vi "CSClassUtilities.TestClass.vi"() -> ()   [LabVIEW 2014]
doc: "Test VI for objects and classes.\n\nLicense Agreement for this software:\n\nCopyright (C) 2001 Dietrich Beck, Holger Brand, Mathias Richter\nGSI Helmholtzzentrum für Schwerionenforschung GmbH\nPlanckstraße 1\nD-64291 Darmstadt\nGermany\n\nContact: d.beck@gsi.de \n\nThis program is free software: you can redistribute it and/or modify it under the terms\nof the GNU General Public License as published by the Free Software Foundation, either\nversion 3 of the License, or (at your option) any later version.\n\nThis program is distributed in the hope that it will be useful, but WITHOUT ANY WARRANTY;\nwithout even the implied warranty of MERCHANTABILITY or FITNESS FOR A PARTICULAR PURPOSE. See the GNU General Public License for more details.\n\nYou should have received a copy of the GNU General Public License along with this program.\nIf not, see <http://www.gnu.org/licenses/>.\n\nFor all questions and ideas contact: d.beck@gsi.de\nLast update: 19-Nov-2010"
uses:
  CSClass/CS_Core/CSSystem/CoreDefs/CoreDefs.error_type.ctl
  CSClass/CS_Core/CSObj/CSObj.lvlib
  CSClass/CS_Core/CSSystem/CoreLib/CoreLib.lvlib
  CSClass/CS_Core/CAEObj/CAEObj.lvlib
  CSClass/CS_Core/NotifierObj/NotifierObj.lvlib
  CSClass/CS_Core/BaseProcess/BaseProcess.lvlib
  CSClass/CS_Core/SuperProc/SuperProc.lvlib
  CSClass/CS_Core/BaseGUI/BaseGUI.lvlib
  CSClass/CS_Core/ObjectInspector/ObjectInspector.lvlib
  CSClass/CS_Core/BaseSM/BaseSM.lvlib
  CSClass/CS_Core/CSSystem/CSSystemLib/CSSystemLib.lvlib
  CSClass/CS_Core/GUIs/GeneralObjectGUI/GeneralObjectGUI.lvlib
  CSClass/CS_Core/CSAccessSystem/CSAccessClient/CSAccessClient.lvlib
  CSClass/CS_Core/GUIs/GOGFrontPanel/GOGFrontPanel.lvlib
panel:
  in  "destroy all objects":bool
  in  "Expert Attr View":bool
  in  "TestProcCases":bool
  in  "Ping":bool
  in  "Object Classes":i32(listbox)=-1
  out "i attribute":variant=variant(cluster{"VI Refnum":refnum<vi>, "Front Panel Ref":refnum<vi>, "semaphore":refnum<k1>, "date of birth":u32} {"VI Refnum"=refnum, "Front Panel Ref"=refnum, "semaphore"=refnum, "date of birth"=511974648})
  out "Error":bool
  in  "Get Attribute":bool
  in  "Select Object":i32(listbox)=-1
  in  "Select Class":i32(listbox)=-1
  out "Error String":string="No Error"
  in  "Close FP":bool
  in  "Open FP":bool
  in  "Destroy":bool
  in  "object name":string
  in  "Create":bool
  in  "Exit":bool
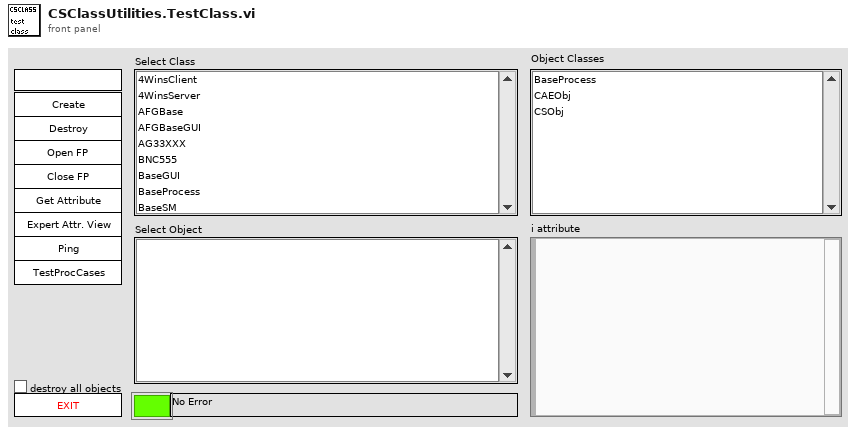
[diagram p1: front panel]
types:
  T1 = enum16{"simple", "synchronous", "asynchronous", "notification"}
  T2 = typedef "CoreDefs.error_type.ctl" = enum16{"no error", "can't load process", "can't unload process", "process does not exist", "can't install process", "can't remove process", "unknown function", "time out", "can't execute function", "duplicate queue name", "super not found", "caller queue invalid", "can't ping process", "unknown error", "VISA Error", "VISA timeout", "GPIB timeout", "GPIB error", "communication error", "data type mismatch", "can't read data from OPC server", "can't write data to OPC server", "OET error", "function not implemented", "process already exists", "invalid Shared Variable name", "error writing Shared Variable", "error reading Shared Variable", "invalid client name", "corrupt database", "unknown class", "call not authorized", "parameter out of range", "OET timeout: can't get data to modify", "invalid queue name", "requested operation incompatible with current state", "event undefined", "event disabled", "state undefined", "caller is not a friend", "EventBuilder: bad eventID", "EventBuilder: no DAQ devices", "a thread must not stop itself", "UNUSED ELEMENT4", "DiscArchiver: eventData incomplete", "DiscArchiver: eventData does not belong to run", "DiscArchiver: can't open file", "DiscArchiver: can't write to file", "DiscArchiver: available disc space low", "can't acquire semaphore", "error reading data from database", "notifier object is not existing", "can't register process", "can't unregister process", "illegal event type", "object disabled", "object already exists", "can't change state", "Instrument not found", "no connection to remote node", "invalid reference", "N/A", "UNUSED ELEMENT 1", "element not found", "illegal TCP/IP connection detected", "object does not exist", "invalid access ID", "unknown CS system", "invalid privilige", "unsupported data type", "unsupported server type", "IO server already exists", "Shared Variable already exists"}
  T3 = typedef "BaseGUI.lvlib/BaseGUI.i attribute.ctl" = cluster{"thread ref":refnum<vi>}
  T4 = typedef "BaseProcess.lvlib/BaseProcess.i attribute.ctl" = cluster{"EventStatus":string, "EventError":i32, "PresetEvtWatchD":i32, "PresetPdcWatchD":i32, "EventTimeout":i32, "PeriodicInterval":i32, "Interface":string[], "Address":string[], "Special":string[], "PeriodicError":i32, "PeriodicStatus":string, "SuperProc":string, "Descriptors":T5[], "CaseRef":refnum<vi>, "PdcRef":refnum<vi>, "Thread Ref":refnum<vi>, "eventErrorID":i32, "eventStatusID":i32, "periodicErrorID":i32, "periodicStatusID":i32, "pdcCtrID":i32}
  T5 = typedef "BaseProcess.lvlib/BaseProcess.descriptor definition.ctl" = cluster{"selector":string, "descriptor":T6}
  T6 = typedef "BaseProcess.lvlib/BaseProcess.descriptor string definition.ctl" = string
  T7 = typedef "BaseSM.lvlib/BaseSM.i attribute.ctl" = cluster{"stateError":i32, "stateStatus":string, "stateQuality":T8, "ProcStateRef":refnum<vi>, "thread ref":refnum<vi>, "actState":string, "reqState":string, "SMQueue":refnum<queue>, "stateErrorID":i32, "stateStatusID":i32}
  T8 = typedef "BaseSM.lvlib/BaseSM.stateQuality.ctl" = i16
  T9 = typedef "CAEObj.lvlib/CAEObj.i attribute.ctl" = cluster{"initialized":bool, "active":bool, "stop":bool, "evtCtrID":i32, "queue":T10, "selector":string[], "URL":string[], "commandID":i32[], "enable":bool[], "ignoreResID":bool[], "NotifyObj":refnum<vi>, "myAccessID":i32, "treeParentName":string, "myAccessIDID":i32, "treeParentAccessIDID":i32, "treeParentNameID":i32, "treeParentAccessIDRef":T11, "treeParentNameRef":T11, "threadRef":refnum<vi>}
  T10 = typedef "LVDimInterface.lvlib/LVDimInterface.queue type.ctl" = refnum<queue>
  T11 = typedef "LVDimInterface.lvlib/LVDimInterface.notifier type.ctl" = refnum<notifier>
  T12 = typedef "CSAccessClient.lvlib/CSAccessClient.i attribute.ctl" = cluster{"creatorRef":refnum<vi>, "actualTreeID":i32, "actualTreeRef":T11}
  T13 = typedef "CSObj.lvlib/CSObj.i attribute.ctl" = cluster{"VI Refnum":refnum<vi>, "Front Panel Ref":refnum<vi>, "semaphore":T14, "date of birth":dbl, "ageID":i32, "systemID":i32, "classID":i32, "conditionID":i32, "DefaultPanelType":u16}
  T14 = typedef "Semaphore RefNum" = refnum<k1>
  T15 = typedef "GeneralObjectGUI.lvlib/GeneralObjectGUI.i attribute.ctl" = cluster{"objects":T16[], "setting file":string, "fpElements":cluster{"busy":refnum<vi>, "status":refnum<vi>}, "accessClientRef":refnum<vi>, "ColumnWidth":u32[], "PanelBounds":T19}
  T16 = typedef "GeneralObjectGUI.lvlib/GeneralObjectGUI.object.ctl" = cluster{"name":string, "systemID":string, "AutoCreate":bool, "Enable":bool, "methods":T17[], "ActError":i32, "Tags":T18[]}
  T17 = typedef "GeneralObjectGUI.lvlib/GeneralObjectGUI.method.ctl" = cluster{"AutoExecute":bool, "Reset":bool, "Enable":bool, "Name":string, "Values":cluster{"descriptor":string, "value":string}[], "fp ref":refnum<vi>}
  T18 = typedef "GeneralObjectGUI.lvlib/GeneralObjectGUI.tag.ctl" = cluster{"name":string, "value":string}
  T19 = typedef "LVRectTypeDef.ctl" = cluster{"Left":i16, "Top":i16, "Right":i16, "Bottom":i16}
  T20 = typedef "GOGFrontPanel.lvlib/GOGFrontPanel.i attribute.ctl" = cluster{"GOGObject":string, "Object":string, "Method":string, "Descriptor":T6, "Input Descriptor":string, "Output Descriptor":string, "inputNames":string[], "outputNames":string[], "Values":cluster{"descriptor":string, "value":string}[]}
  T21 = typedef "NotifierObj.lvlib/NotifierObj.i attribute.ctl" = cluster{"associatedObjRef":refnum<vi>, "Notifiers":cluster{"Name":string, "Message":i8[], "Noti missed":i32, "Msg Sent":bool, "ref":T11}[], "commandIDs":i32[], "request stop":bool, "thread ref":refnum<vi>, "Enqueue at opposite":bool}
  T22 = typedef "ObjectInspector.lvlib/ObjectInspector.i attribute.ctl" = cluster{"ClassPaths":string[]}
  T23 = typedef "SuperProc.lvlib/SuperProc.i attribute.ctl" = cluster{"Proc Tbl":T24[]}
  T24 = typedef "SuperProc.lvlib/SuperProc.proc_tbl_type.ctl" = cluster{"Name":string, "Connections":i32, "Clients":string[], "EvtWDAlarmTime":u32, "PdcWDAlarmTime":u32, "PresetEvtWatchD":i32, "PresetPdcWatchD":i32, "i ref":refnum<vi>, "evtCounterRef":T11, "evtCounterID":i32, "pdcCounterRef":T11, "pdcCounterID":i32, "watchdogValue":i32, "watchdogID ":i32}
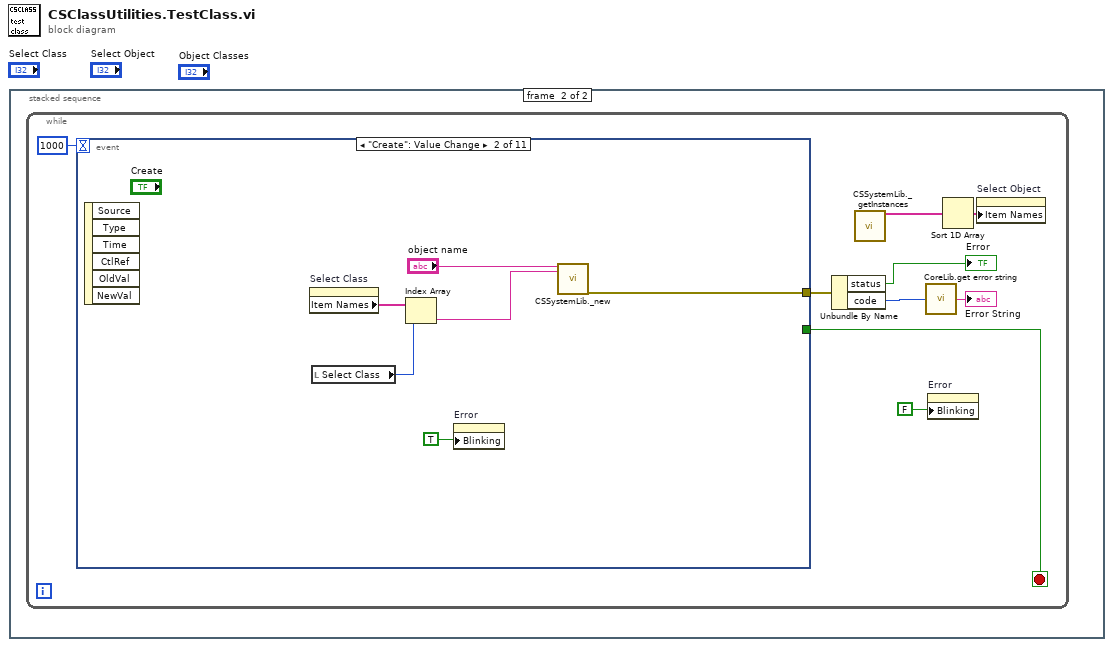
[diagram p0: block diagram]
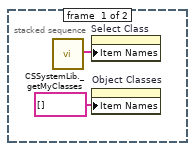
[diagram p2: hidden frame]
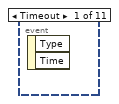
[diagram p3: hidden frame]
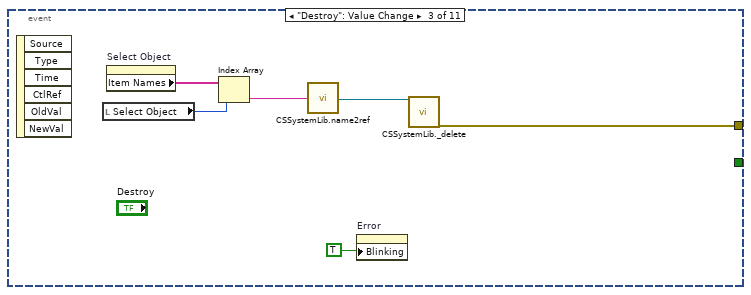
[diagram p4: hidden frame]
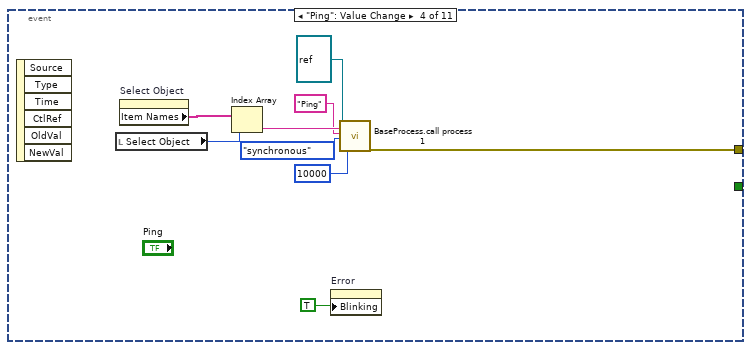
[diagram p5: hidden frame]
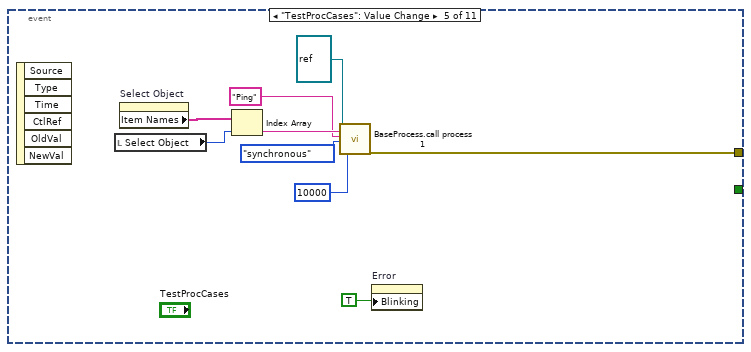
[diagram p6: hidden frame]
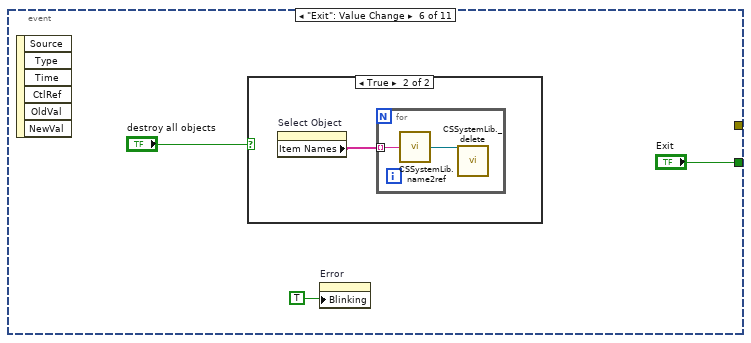
[diagram p7: hidden frame]
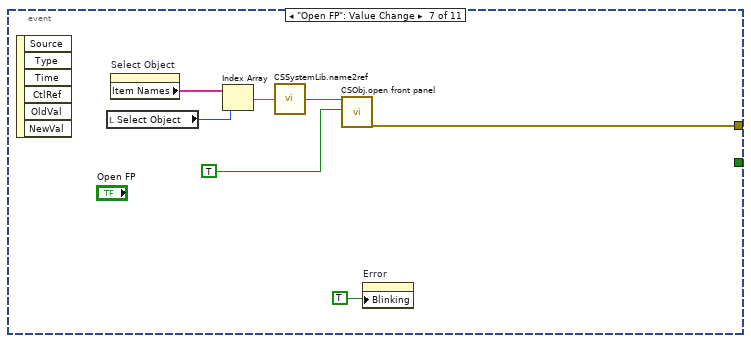
[diagram p9: hidden frame]
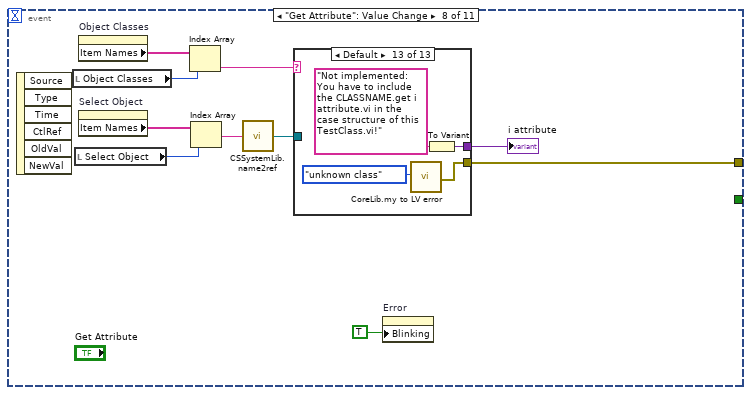
[diagram p10: hidden frame]
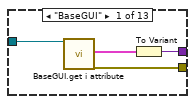
[diagram p11: hidden frame]
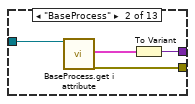
[diagram p12: hidden frame]
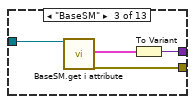
[diagram p13: hidden frame]
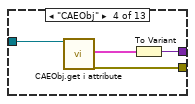
[diagram p14: hidden frame]
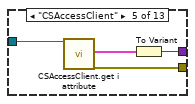
[diagram p15: hidden frame]
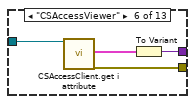
[diagram p16: hidden frame]
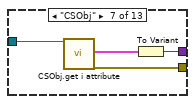
[diagram p17: hidden frame]
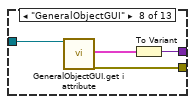
[diagram p18: hidden frame]
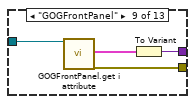
[diagram p19: hidden frame]
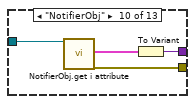
[diagram p20: hidden frame]
diagram:
  n1 = stacked-sequence {
    frame #0 {
      n2 = call "CSSystemLib._getMyClasses.vi"() -> ("myClasses"=w2:string[])  [unwired: 18 in, 1 out]
      n3 = property on="Select Class" class="LstBox (strict)"("Item Names"=w2) -> ()  [unwired: 2 in, 2 out]
      n4 = property on="Object Classes" class="LstBox (strict)"("Item Names"=string[] []) -> ()  [unwired: 2 in, 2 out]
    }
    frame #1 {
      n5 = while {
        stop <- w11 stop-if-true
        n6 = event shown="[1] \"Create\": Value Change" {
          selector: _ -> [_ _ _ _ _ _ _ _ _ _ _]
          dyn-events: _ -> [_ _ _ _ _ _ _ _ _ _ _]
          timeout: 1000 -> [_ _ _ _ _ _ _ _ _ _ _]
          tunnel: [_ _ _ _ _ "Exit" _ _ _ _ _] -> w11
          tunnel: [_ w16 w22 w26 w35 _ w52 w57 _ w133 _] -> w8
          event Timeout {
            n7 = event-data() -> ()  [unwired: 1 in, 2 out]
          }
          event "Create": Value Change {
            n8 = event-data() -> ()  [unwired: 1 in, 6 out]
            n9 = property on="Select Class" class="LstBox (strict)"() -> ("Item Names"=w15:string[])  [unwired: 2 in, 2 out]
            n10 = local read "Select Class"() -> (w14:i32)
            n11 = Index Array(array=w15, index=w14) -> (element=w13:string)
            n12 = property on="Error" class="Bool (strict)"("Blinking"=TRUE) -> ()  [unwired: 2 in, 2 out]
            n13 = call "CSSystemLib._new.vi"("object name"="object name", "class name"=w13) -> ("error out"=w16:errorcluster)  [unwired: 14 in, 3 out]
          }
          event "Destroy": Value Change {
            n14 = event-data() -> ()  [unwired: 1 in, 6 out]
            n15 = local read "Select Object"() -> (w20:i32)
            n16 = property on="Select Object" class="LstBox (strict)"() -> ("Item Names"=w21:string[])  [unwired: 2 in, 2 out]
            n17 = Index Array(array=w21, index=w20) -> (element=w19:string)
            n18 = call "CSSystemLib.name2ref.vi"("name"=w19) -> ("obj refnum"=w23:refnum<vi>)
            n19 = property on="Error" class="Bool (strict)"("Blinking"=TRUE) -> ()  [unwired: 2 in, 2 out]
            n20 = call "CSSystemLib._delete.vi"("i ref"=w23) -> ("error out"=w22:errorcluster)  [unwired: 18 in]
          }
          event "Ping": Value Change {
            n21 = event-data() -> ()  [unwired: 1 in, 6 out]
            n22 = local read "Select Object"() -> (w32:i32)
            n23 = property on="Select Object" class="LstBox (strict)"() -> ("Item Names"=w31:string[])  [unwired: 2 in, 2 out]
            n24 = Index Array(array=w31, index=w32) -> (element=w30:string)
            n25 = property on="Error" class="Bool (strict)"("Blinking"=TRUE) -> ()  [unwired: 2 in, 2 out]
            n26 = call "BaseProcess.call process 1.vi"("i ref in"=refnum<vi> refnum, "Object"=w30, "Selector"="Ping", "CallType"=T1."synchronous", "timeout (ms)"=10000) -> ("error out"=w26:errorcluster)  [unwired: 12 in, 2 out]
          }
          event "TestProcCases": Value Change {
            n27 = event-data() -> ()  [unwired: 1 in, 6 out]
            n28 = local read "Select Object"() -> (w41:i32)
            n29 = property on="Select Object" class="LstBox (strict)"() -> ("Item Names"=w40:string[])  [unwired: 2 in, 2 out]
            n30 = Index Array(array=w40, index=w41) -> (element=w39:string)
            n31 = call "BaseProcess.call process 1.vi"("i ref in"=refnum<vi> refnum, "Object"=w39, "Selector"="Ping", "CallType"=T1."synchronous", "timeout (ms)"=10000) -> ("error out"=w35:errorcluster)  [unwired: 12 in, 2 out]
            n32 = property on="Error" class="Bool (strict)"("Blinking"=TRUE) -> ()  [unwired: 2 in, 2 out]
          }
          event "Exit": Value Change {
            n33 = event-data() -> ()  [unwired: 1 in, 6 out]
            n34 = case shown="True" "destroy all objects" {
              frame False {
              }
              frame True {
                n35 = property on="Select Object" class="LstBox (strict)"() -> ("Item Names"=w45:string[])  [unwired: 2 in, 2 out]
                n36 = for {
                  tunnel: w45 -> [w47] mode=indexing
                  n37 = call "CSSystemLib.name2ref.vi"("name"=w47) -> ("obj refnum"=w46:refnum<vi>)
                  n38 = call "CSSystemLib._delete.vi"("i ref"=w46) -> ()  [unwired: 18 in, 1 out]
                }
              }
            }
            n39 = property on="Error" class="Bool (strict)"("Blinking"=TRUE) -> ()  [unwired: 2 in, 2 out]
          }
          event "Open FP": Value Change {
            n40 = event-data() -> ()  [unwired: 1 in, 6 out]
            n41 = local read "Select Object"() -> (w49:i32)
            n42 = property on="Select Object" class="LstBox (strict)"() -> ("Item Names"=w51:string[])  [unwired: 2 in, 2 out]
            n43 = Index Array(array=w51, index=w49) -> (element=w50:string)
            n44 = call "CSSystemLib.name2ref.vi"("name"=w50) -> ("obj refnum"=w54:refnum<vi>)
            n45 = call "CSObj.open front panel.vi"("i ref in"=w54, "frontPanelOpen"=TRUE ("front panel open")) -> ("error out"=w52:errorcluster)  [unwired: 16 in, 1 out]
            n46 = property on="Error" class="Bool (strict)"("Blinking"=TRUE) -> ()  [unwired: 2 in, 2 out]
          }
          event "Get Attribute": Value Change {
            n47 = event-data() -> ()  [unwired: 1 in, 6 out]
            n48 = local read "Object Classes"() -> (w60:i32)
            n49 = local read "Select Object"() -> (w62:i32)
            n50 = property on="Object Classes" class="LstBox (strict)"() -> ("Item Names"=w61:string[])  [unwired: 2 in, 2 out]
            n51 = property on="Select Object" class="LstBox (strict)"() -> ("Item Names"=w64:string[])  [unwired: 2 in, 2 out]
            n52 = Index Array(array=w61, index=w60) -> (element=w59:string)
            n53 = Index Array(array=w64, index=w62) -> (element=w63:string)
            n54 = call "CSSystemLib.name2ref.vi"("name"=w63) -> ("obj refnum"=w58:refnum<vi>)
            n55 = case shown="Default" w59 {
              tunnel: w58 -> [w68 w72 w76 w80 w84 w88 w92 w96 w100 w104 w108 w112 _]
              tunnel: [w65 w69 w73 w77 w81 w85 w90 w93 w97 w102 w105 w109 w114] -> w56
              tunnel: [w67 w71 w75 w79 w83 w87 w91 w95 w99 w103 w107 w111 w115] -> w57
              frame "BaseGUI" {
                n56 = call "BaseGUI.get i attribute.vi"("i ref in"=w68) -> ("i attribute"=w66:T3, "error out"=w67:errorcluster)  [unwired: 16 in, 1 out]
                n57 = To Variant(anything=w66) -> (Variant=w65:variant)
              }
              frame "BaseProcess" {
                n58 = call "BaseProcess.get i attribute.vi"("i ref in"=w72) -> ("i attribute"=w70:T4, "error out"=w71:errorcluster)  [unwired: 16 in, 1 out]
                n59 = To Variant(anything=w70) -> (Variant=w69:variant)
              }
              frame "BaseSM" {
                n60 = call "BaseSM.get i attribute.vi"("i ref in"=w76) -> ("i attribute"=w74:T7, "error out"=w75:errorcluster)  [unwired: 16 in, 1 out]
                n61 = To Variant(anything=w74) -> (Variant=w73:variant)
              }
              frame "CAEObj" {
                n62 = call "CAEObj.get i attribute.vi"("i ref in"=w80) -> ("i attribute"=w78:T9, "error out"=w79:errorcluster)  [unwired: 16 in, 1 out]
                n63 = To Variant(anything=w78) -> (Variant=w77:variant)
              }
              frame "CSAccessClient" {
                n64 = call "CSAccessClient.get i attribute.vi"("i ref in"=w84) -> ("i attribute"=w82:T12, "error out"=w83:errorcluster)  [unwired: 16 in, 1 out]
                n65 = To Variant(anything=w82) -> (Variant=w81:variant)
              }
              frame "CSAccessViewer" {
                n66 = call "CSAccessClient.get i attribute.vi"("i ref in"=w88) -> ("i attribute"=w86:T12, "error out"=w87:errorcluster)  [unwired: 16 in, 1 out]
                n67 = To Variant(anything=w86) -> (Variant=w85:variant)
              }
              frame "CSObj" {
                n68 = call "CSObj.get i attribute.vi"("i ref in"=w92) -> ("i attribute"=w89:T13, "error out"=w91:errorcluster)  [unwired: 16 in, 1 out]
                n69 = To Variant(anything=w89) -> (Variant=w90:variant)
              }
              frame "GeneralObjectGUI" {
                n70 = call "GeneralObjectGUI.get i attribute.vi"("i ref in"=w96) -> ("i attribute"=w94:T15, "error out"=w95:errorcluster)  [unwired: 16 in, 1 out]
                n71 = To Variant(anything=w94) -> (Variant=w93:variant)
              }
              frame "GOGFrontPanel" {
                n72 = call "GOGFrontPanel.get i attribute.vi"("i ref in"=w100) -> ("i attribute"=w98:T20, "error out"=w99:errorcluster)  [unwired: 16 in, 1 out]
                n73 = To Variant(anything=w98) -> (Variant=w97:variant)
              }
              frame "NotifierObj" {
                n74 = call "NotifierObj.get i attribute.vi"("i ref in"=w104) -> ("i attribute"=w101:T21, "error out"=w103:errorcluster)  [unwired: 16 in, 1 out]
                n75 = To Variant(anything=w101) -> (Variant=w102:variant)
              }
              frame "ObjectInspector" {
                n76 = call "ObjectInspector.get i attribute.vi"("i ref in"=w108) -> ("i attribute"=w106:T22, "error out"=w107:errorcluster)  [unwired: 16 in, 1 out]
                n77 = To Variant(anything=w106) -> (Variant=w105:variant)
              }
              frame "SuperProc" {
                n78 = call "SuperProc.get i attribute.vi"("i ref in"=w112) -> ("i attribute"=w110:T23, "error out"=w111:errorcluster)  [unwired: 16 in, 1 out]
                n79 = To Variant(anything=w110) -> (Variant=w109:variant)
              }
              frame Default {
                n80 = call "CoreLib.my to LV error.vi"("ErrorTypes"=CoreDefs.error_type."unknown class") -> ("myErrorCluster"=w115:errorcluster)  [unwired: 17 in, 1 out]
                n81 = To Variant(anything="Not implemented: You have to include the CLASSNAME.get i attribute.vi in the case structure of this TestClass.vi!" ("xml string")) -> (Variant=w114:variant)
              }
            }
            "i attribute" <- w56
            n82 = property on="Error" class="Bool (strict)"("Blinking"=TRUE) -> ()  [unwired: 2 in, 2 out]
          }
          event "Expert Attr View": Value Change {
            n83 = event-data() -> ()  [unwired: 1 in, 6 out]
            n84 = local read "Object Classes"() -> (w127:i32)
            n85 = property on="Object Classes" class="LstBox (strict)"() -> ("Item Names"=w128:string[])  [unwired: 2 in, 2 out]
            n86 = Index Array(array=w128, index=w127) -> (element=w120:string)
            n87 = property on="Error" class="Bool (strict)"("Blinking"=TRUE) -> ()  [unwired: 2 in, 2 out]
            n88 = Concatenate Strings(w120, ".lvlib:" ("string"), w120, ".get i attribute.vi" ("string")) -> (w125:string)
            n89 = Open VI Reference(vi path=w125) -> (vi reference=w124:refnum<vi>, error out=w118:errorcluster)  [unwired: 5 in]
            n90 = property on="Property Node" class="VI"(reference=w124, error in=w118, "Front Panel Window:Open"=TRUE) -> (reference out=w122:refnum<vi>, error out=w117:errorcluster)
            n91 = Close Reference(reference=w122, error in (no error)=w117) -> ()  [unwired: 1 out]
          }
          event "Close FP": Value Change {
            n92 = event-data() -> ()  [unwired: 1 in, 6 out]
            n93 = local read "Select Object"() -> (w131:i32)
            n94 = property on="Select Object" class="LstBox (strict)"() -> ("Item Names"=w132:string[])  [unwired: 2 in, 2 out]
            n95 = Index Array(array=w132, index=w131) -> (element=w130:string)
            n96 = call "CSSystemLib.name2ref.vi"("name"=w130) -> ("obj refnum"=w135:refnum<vi>)
            n97 = call "CSObj.open front panel.vi"("i ref in"=w135, "frontPanelOpen"=FALSE ("front panel open")) -> ("error out"=w133:errorcluster)  [unwired: 16 in, 1 out]
            n98 = property on="Error" class="Bool (strict)"("Blinking"=TRUE) -> ()  [unwired: 2 in, 2 out]
          }
          event "Select Object": Value Change {
            n99 = event-data() -> ("NewVal"=w139:i32)  [unwired: 1 in, 5 out]
            n100 = property on="Select Object" class="LstBox (strict)"() -> ("Item Names"=w141:string[])  [unwired: 2 in, 2 out]
            n101 = Index Array(array=w141, index=w139) -> (element=w138:string)
            n102 = property on="Error" class="Bool (strict)"("Blinking"=TRUE) -> ()  [unwired: 2 in, 2 out]
            n103 = call "CSSystemLib.name2ref.vi"("name"=w138) -> ("obj refnum"=w136:refnum<vi>)
            n104 = call "CSSystemLib.ref2classNames.vi"("obj refnum"=w136) -> ("classNames"=w137:string[])
            n105 = property on="Object Classes" class="LstBox (strict)"("Item Names"=w137) -> ()  [unwired: 2 in, 2 out]
          }
        }
        n106 = Unbundle By Name(w8) -> ("status"=→"Error":bool, "code"=w10:i32)
        n107 = call "CSSystemLib._getInstances.vi"() -> ("i list"=w3:string[])  [unwired: 18 in, 1 out]
        n108 = call "CoreLib.get error string.vi"("Error Code"=w10) -> ("Error String"=→"Error String":string)
        n109 = property on="Error" class="Bool (strict)"("Blinking"=FALSE) -> ()  [unwired: 2 in, 2 out]
        n110 = Sort 1D Array(array=w3) -> (sorted array=w5:string[])
        n111 = property on="Select Object" class="LstBox (strict)"("Item Names"=w5) -> ()  [unwired: 2 in, 2 out]
      }
    }
  }
